vi "Compute amplitudes.vi"(11 "Run amplitude bundle":T1={"# of amplitudes"=1, "Amplitude type?"=0, "Amplitude 1"=3.0, "step size"=0.0, "Amplitude array"=[]} {"step size" format="%.2f"; "Amplitude 1" min=-10.0 max=10.0 format="%.2f"; "Amplitude type?" items=["Linear", "Array"]}) -> (3 "Amplitudes":dbl[](array[numeric]))   [LabVIEW 2010]
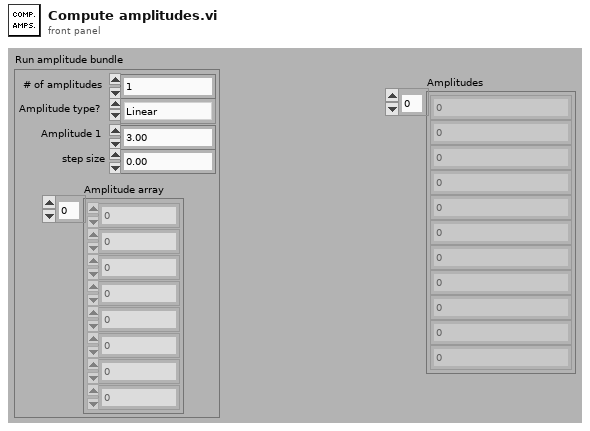
[diagram p1: front panel]
types:
  T1 = cluster{"# of amplitudes":i32, "Amplitude type?":u16, "Amplitude 1":dbl, "step size":dbl, "Amplitude array":dbl[]}
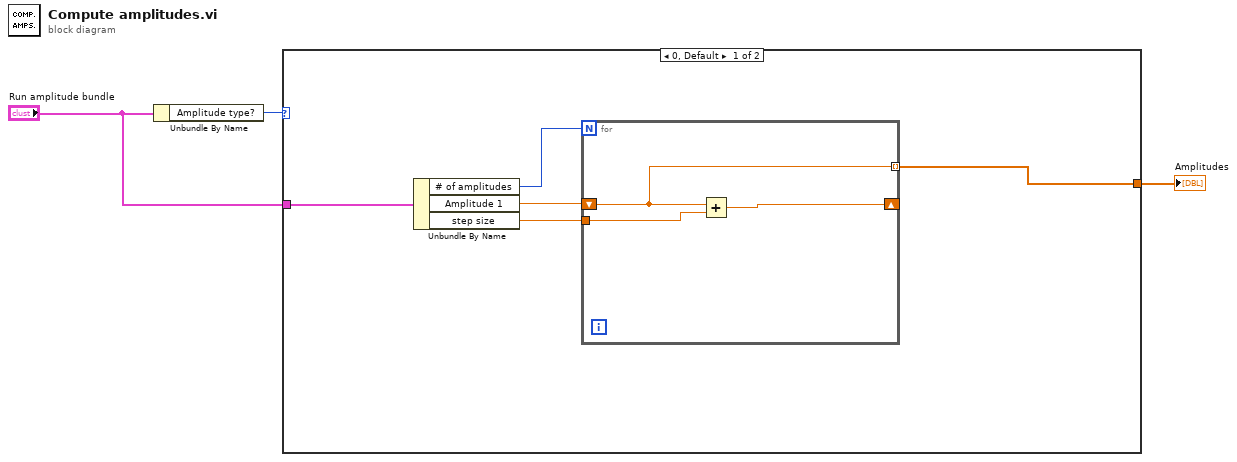
[diagram p0: block diagram]
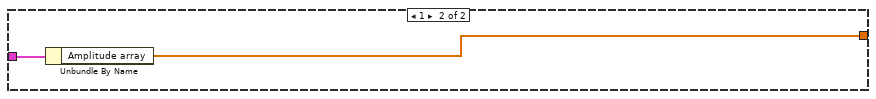
[diagram p2: hidden frame]
diagram:
  n1 = Unbundle By Name("Run amplitude bundle") -> ("Amplitude type?"=w3:u16)
  n2 = case shown="0, Default" w3 {
    tunnel: "Run amplitude bundle" -> [w8 w13]
    tunnel: [w4 w12] -> w1
    frame 0, Default {
      n3 = Unbundle By Name(w8) -> ("# of amplitudes"=w7:i32, "Amplitude 1"=w6:dbl, "step size"=w5:dbl)
      n4 = for {
        N: w7 -> [_]
        shift-right: [w10] -> _
        shift-left: w6 -> [w9]
        tunnel: w5 -> [w11]
        tunnel: [w9] -> w4 mode=indexing
        n5 = Add(x=w9, y=w11) -> (x+y=w10:dbl)
      }
    }
    frame 1 {
      n6 = Unbundle By Name(w13) -> ("Amplitude array"=w12:dbl[])
    }
  }
  "Amplitudes" <- w1
